vi "AverageReplicates.vi"(9 "setup":T1={"# replicates"=5, "Sample time (msec)"=5, "Motor Steps"=5}, 10 "Data set":string) -> (0 "measured angles":cluster{i32, dbl, dbl[]}[](graph), 3 "Normalized angles":cluster{i32, dbl, dbl[]}[](graph), 4 "All lines":cluster{i32, dbl, dbl[]}[](graph))   [LabVIEW 2022 SP3]
panel:
  # "1. How many times do you want to run the same speed"
  # "2. millisec between data points (1/sampling rate)?"
  # "3. Run motor speeds from 0 to 100 in steps of?"
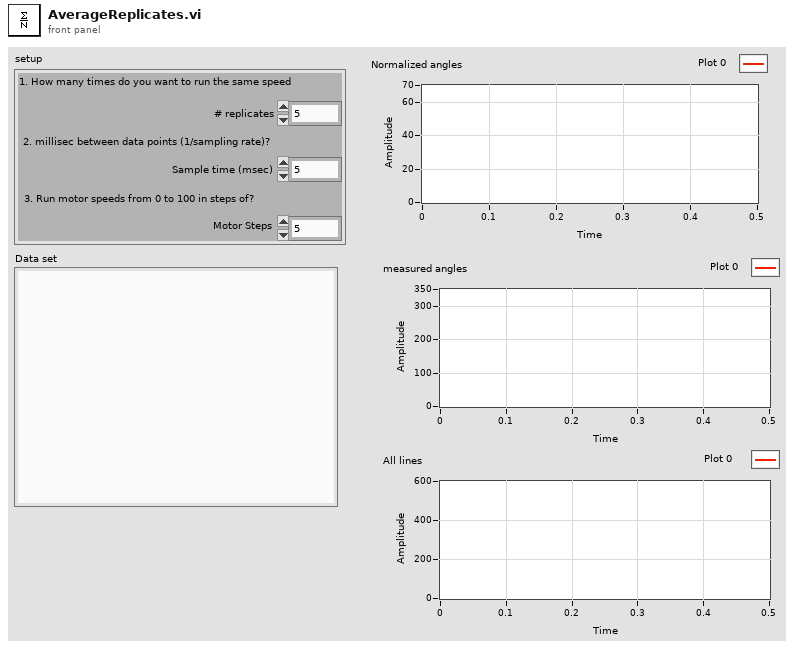
[diagram p1: front panel]
types:
  T1 = cluster{"# replicates":i8, "Sample time (msec)":i8, "Motor Steps":i8}
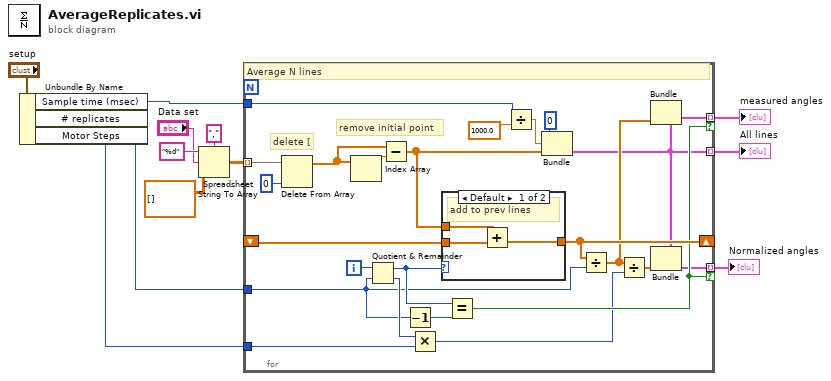
[diagram p0: block diagram]
diagram:
  n1 = Unbundle By Name("setup") -> ("Sample time (msec)"=w3:i8, "# replicates"=w2:i8, "Motor Steps"=w1:i8)
  n2 = Spreadsheet String To Array(delimiter (Tab)=",", format string="%d", spreadsheet string="Data set", array type (2D Dbl)=dbl[][] []) -> (array=w9:dbl[][])
  n3 = for {
    tunnel: w9 -> [w35] mode=indexing
    tunnel: [w19] -> w10 mode=indexing
    shift-right: [w31] -> _
    shift-left: _ -> [w32]
    tunnel: [w18] -> w11 mode=indexing if=w26
    tunnel: [w21] -> w12 mode=indexing if=w26
    tunnel: w1 -> [w25]
    tunnel: w2 -> [w16]
    tunnel: w3 -> [w15]
    i -> [w28]
    # "remove initial point"
    # "delete ["
    # "Average N lines"
    n4 = Delete From Array(array=w35, index=0) -> (array with subset deleted=w33:dbl[])  [unwired: 1 in, 1 out]
    n5 = Index Array(array=w33) -> (element=w36:dbl)  [unwired: 1 in]
    n6 = Quotient & Remainder(x=w28, y=w16) -> (x-y*floor(x/y)=w29:i32, floor(x/y)=w27:i32)
    n7 = Subtract(x=w33, y=w36) -> (x-y=w24:dbl[])
    n8 = Decrement(x=w16) -> (x-1=w30:i8)
    n9 = Multiply(x=w27, y=w25) -> (x*y=w17:i32)
    n10 = case shown="Default" w29 {
      tunnel: [w37 w40] -> w31
      tunnel: w24 -> [w39 w40]
      tunnel: w32 -> [w38 _]
      frame Default {
        # "add to prev lines"
        n11 = Add(x=w39, y=w38) -> (x+y=w37:dbl[])
      }
      frame 0 {
        # "start of new average"
      }
    }
    n12 = Equal?(x=w29, y=w30) -> (x = y?=w26:bool)
    n13 = Divide(x=w15, y=1000.0) -> (x/y=w13:dbl)
    n14 = Bundle(0, w13, w24) -> (w19:cluster{i32, dbl, dbl[]})  [unwired: 1 in]
    n15 = Divide(x=w31, y=w16) -> (x/y=w22:dbl[])
    n16 = Divide(x=w22, y=w17) -> (x/y=w20:dbl[])
    n17 = Bundle(cluster=w19, w22) -> (w21:cluster{i32, dbl, dbl[]})  [unwired: 2 in]
    n18 = Bundle(cluster=w19, w20) -> (w18:cluster{i32, dbl, dbl[]})  [unwired: 2 in]
  }
  "measured angles" <- w12
  "Normalized angles" <- w11
  "All lines" <- w10
